vi "InitializeUDL.vi"(6 "Parameters":T2={"number of planes"=4, "z step"=1.9999999999999998e-05, "pixel dwell time"=1.0000000000000001e-11, "z frequency"=10.0, "number of pixels"=100, "smooth points"=10, "smooth line"=10, "Sine\nSawtooth"=FALSE, "PointSorting"=0, "Sort Points"=FALSE, "X-pixels"=256.0, "Y-lines"=256.0, "pixelstoµm"=256.0, "zoom"=1.0, "Time offset"=1.0000000000000001e-11} {"zoom" min=0.5 step=0.1; "Y-lines" min=1 step=1; "X-pixels" min=1 step=1; "PointSorting" items=["No Difference", "Every Second Point", "Down / Up"]; "smooth line" min=1; "smooth points" min=1; "number of pixels" min=1; "z frequency" format="%_4g"; "number of planes" min=1}, 8 "error in (no error)":errorcluster, 9 "DutyCluster":T1 {"Iteration" items=["first iteration", "second iteration"]}, 10 "XYZ Point coordinates smoothed (pixels)":dbl[][](array[numeric]), 11 "XYZ Point coordinates selected (pixels)":dbl[][](array[numeric])) -> (0 "error out":errorcluster, 2 "DutyCluster":T1 {"Iteration" items=["first iteration", "second iteration"]}, 3 "XYZ Point coordinates (um)":dbl[][](array[numeric]))   [LabVIEW 2010]
uses:
  TypeDefs/ParameterCluster.ctl
  TypeDefs/DutyCluster.ctl
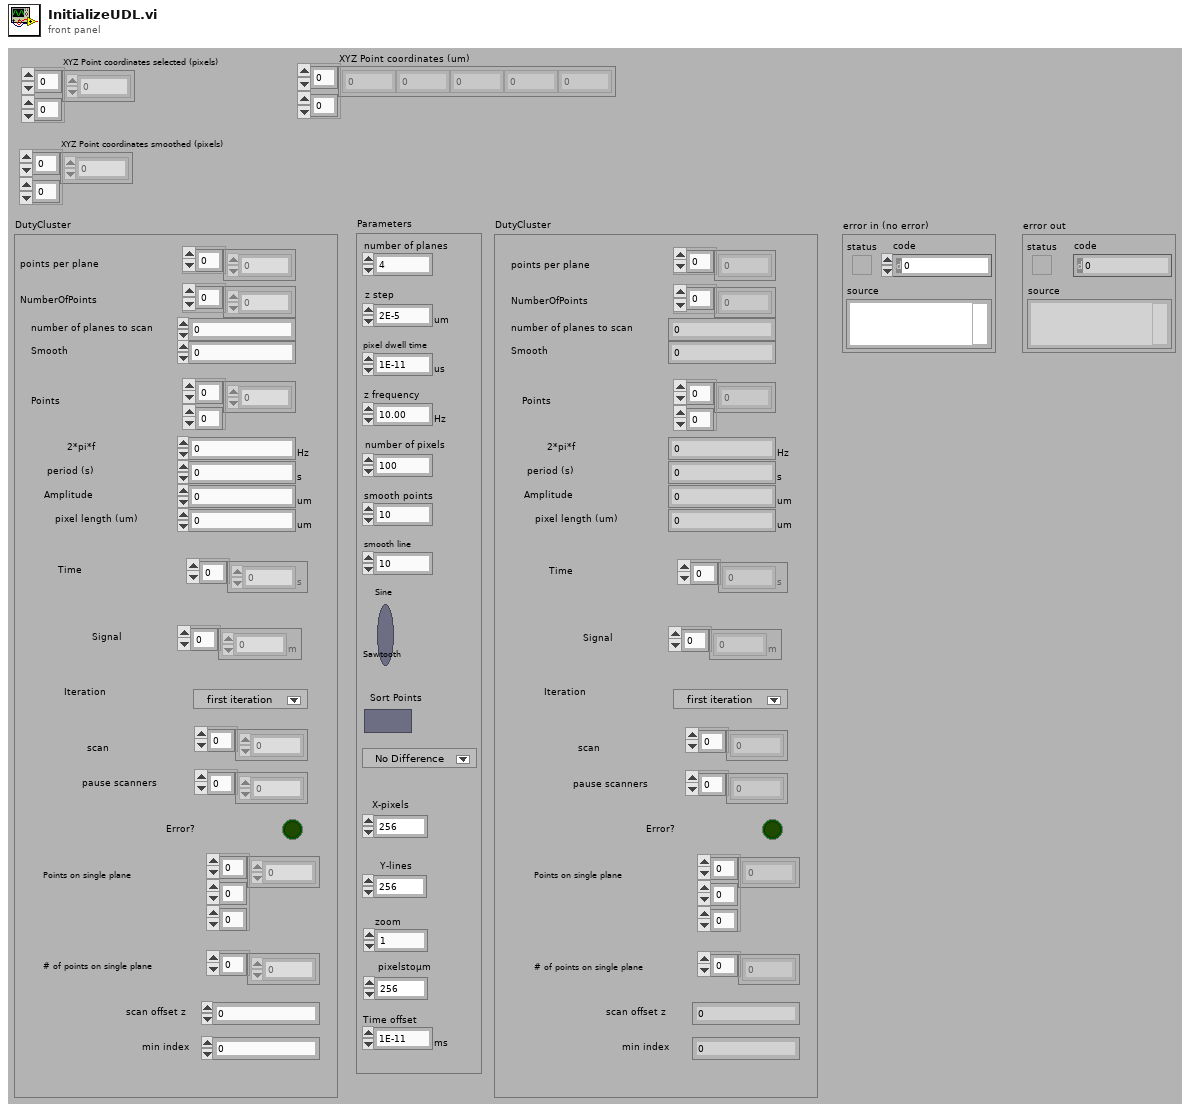
[diagram p1: front panel]
types:
  T1 = typedef "DutyCluster.ctl" = cluster{"points per plane":i32[], "NumberOfPoints":i32[], "number of planes to scan":i32, "Smooth":i32, "Points":dbl[][], "2*pi*f":dbl[unit], "period (s)":dbl[unit], "Amplitude":dbl[unit], "pixel length (um)":dbl[unit], "Time":dbl[unit][], "Signal":dbl[unit][], "Iteration":u16, "scan":i32[], "pause scanners":i32[], "Error?":bool, "Points on single plane":dbl[][][], "# of points on single plane":i32[], "scan offset z":i32, "min index":i32}
  T2 = typedef "ParameterCluster.ctl" = cluster{"number of planes":i32, "z step":dbl[unit], "pixel dwell time":dbl[unit], "z frequency":dbl[unit], "number of pixels":i32, "smooth points":i32, "smooth line":i32, "Sine\nSawtooth":bool, "PointSorting":u16, "Sort Points":bool, "X-pixels":sgl, "Y-lines":sgl, "pixelstoµm":dbl, "zoom":dbl, "Time offset":dbl[unit]}
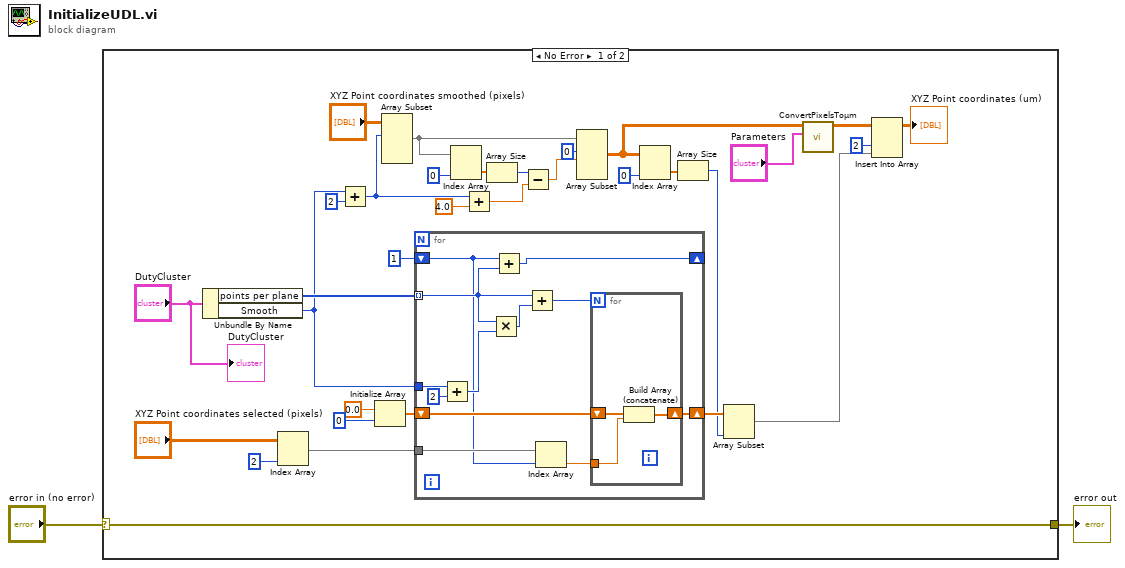
[diagram p0: block diagram]
diagram:
  n1 = case shown="No Error" "error in (no error)" {
    selector: "error in (no error)" -> [w4 w50]
    tunnel: [w4 w50] -> w1
    frame No Error {
      n2 = Unbundle By Name("DutyCluster") -> ("points per plane"=w14:i32[], "Smooth"=w13:i32)
      n3 = Index Array(array="XYZ Point coordinates selected (pixels)", index (col)=2 ("index")) -> (element=w21:dbl[])  [unwired: 1 in]
      n4 = Add(x=w13, y=2) -> (x+y=w24:i32)
      n5 = Initialize Array(0.0 ("element"), 0 ("dimension size")) -> (w17:dbl[])
      n6 = Array Subset(array="XYZ Point coordinates smoothed (pixels)", index (row)=w24) -> (w23:dbl[][])  [unwired: 3 in]
      n7 = for {
        tunnel: w14 -> [w38] mode=indexing
        tunnel: w13 -> [w46]
        tunnel: w21 -> [w42]
        shift-right: [w39] -> w12
        shift-left: w17 -> [w40]
        shift-right: [w37] -> _
        shift-left: 1 -> [w36]
        n8 = Add(x=w46, y=2) -> (x+y=w44:i32)
        n9 = Multiply(x=w38, y=w44) -> (x*y=w43:i32)
        n10 = Add(x=w36, y=w38) -> (x+y=w37:i32)
        n11 = Add(x=w38, y=w43) -> (x+y=w35:i32)
        n12 = Index Array(array=w42, index=w36) -> (element=w41:dbl)
        n13 = for {
          N: w35 -> [_]
          shift-right: [w48] -> w39
          shift-left: w40 -> [w49]
          tunnel: w41 -> [w47]
          n14 = Build Array (concatenate)(w49, w47) -> (w48:dbl[])
        }
      }
      n15 = Index Array(array=w23, index (col)=0 ("disabled index (col)")) -> (element=w32:dbl[])  [unwired: 1 in]
      n16 = Add(x=w24, y=4.0) -> (x+y=w27:dbl)
      n17 = Array Size(array=w32) -> (size(s)=w30:i32)
      n18 = Subtract(x=w30, y=w27) -> (x-y=w28:dbl)
      n19 = Array Subset(array=w23, index (row)=0 ("index"), length (row)=w28) -> (w7:dbl[][])  [unwired: 2 in]
      n20 = Index Array(array=w7, index (col)=0 ("disabled index (col)")) -> (element=w33:dbl[])  [unwired: 1 in]
      n21 = Array Size(array=w33) -> (size(s)=w11:i32)
      n22 = Array Subset(array=w12, length=w11) -> (w8:dbl[])  [unwired: 1 in]
      n23 = call "ConvertPixelsToµm.vi"("Parameters"="Parameters", "Point coordinates (pixels)"=w7) -> ("Point coordinates (µm)"=w9:dbl[][])  [unwired: 6 in, 1 out]
      n24 = Insert Into Array(array=w9, index (col)=2 ("disabled index (col)"), new element=w8) -> (→"XYZ Point coordinates (um)":dbl[][])  [unwired: 1 in]
      "DutyCluster" <- "DutyCluster"
    }
    frame Error {
    }
  }
  "error out" <- w1
